vi "STD获取温度校准参数.vi"(7 "探头":T1(ring), 8 "error in (no error)":errorcluster caption="错误输入（无错误）", 11 "MB session in":refnum<class "MB_Master.lvclass">) -> (0 "error out":errorcluster caption="错误输出", 2 "输出值":cluster{"K":sgl, "B":sgl}, 3 "MB session out":refnum<class "MB_Master.lvclass">)   [LabVIEW 2016, in "斯坦道多参数.lvlib"]
uses:
  <vilib>/Plasmionique/MB Master/MB_Master/MB_Master.lvclass
  <vilib>/Plasmionique/MB Master/MB Master.lvlib
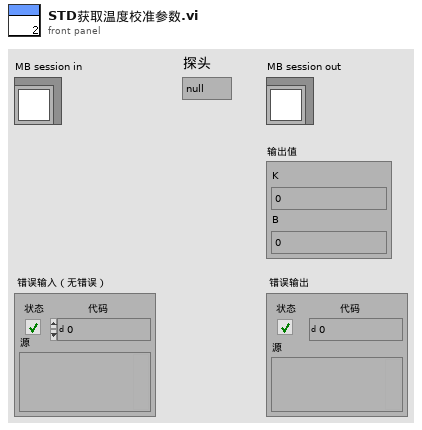
[diagram p1: front panel]
types:
  T1 = enum16{"null", "pH", "DO", "浊度", "电导率", "叶绿素a", "DO2", "藻密度", "悬浮物"}
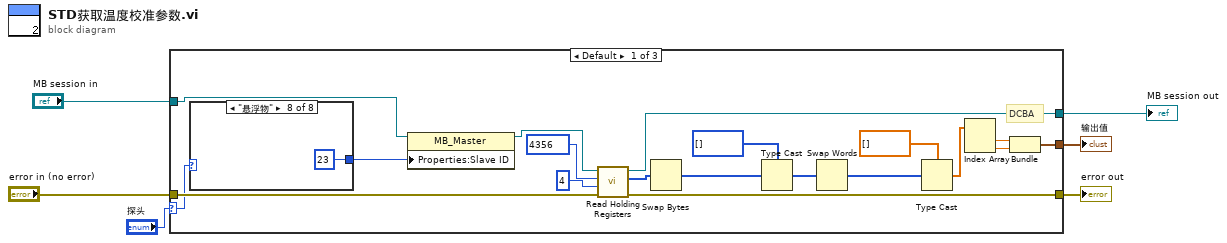
[diagram p0: block diagram]
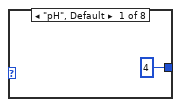
[diagram p2: hidden frame]
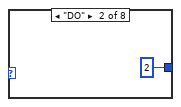
[diagram p3: hidden frame]
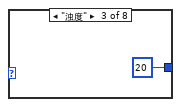
[diagram p4: hidden frame]
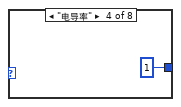
[diagram p5: hidden frame]
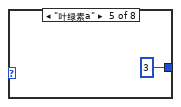
[diagram p6: hidden frame]
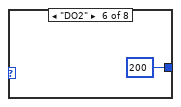
[diagram p7: hidden frame]
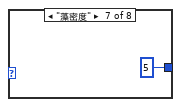
[diagram p8: hidden frame]
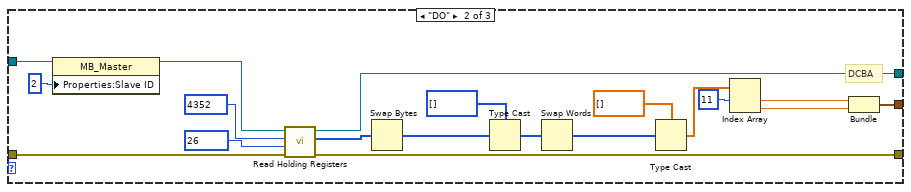
[diagram p9: hidden frame]
diagram:
  n1 = case shown="Default" "探头" {
    selector: "探头" -> [w9 _ _]
    tunnel: "error in (no error)" -> [w16 w43 w53]
    tunnel: [w14 w41 w53] -> w5
    tunnel: "MB session in" -> [w12 w39 w54]
    tunnel: [w11 w38 w54] -> w3
    tunnel: [w8 w36 _] -> w1
    frame Default {
      # "DCBA"
      n2 = case shown="\"悬浮物\"" w9 {
        tunnel: [u16 4 ("y") u16 2 ("y") u16 20 ("y") u16 1 ("y") u16 3 ("y") u16 200 ("y") u16 5 ("y") u16 23 ("y")] -> w10
        frame "pH", Default {
        }
        frame "DO" {
        }
        frame "浊度" {
        }
        frame "电导率" {
        }
        frame "叶绿素a" {
        }
        frame "DO2" {
        }
        frame "藻密度" {
        }
        frame "悬浮物" {
        }
      }
      n3 = property class="MB_Master"(reference=w12, "Properties:Slave ID"=w10) -> (reference out=w15:refnum<class "MB_Master.lvclass">)  [unwired: 1 in, 1 out]
      n4 = call <vilib>:"Read Holding Registers.vi"("error in (no error)"=w16, "quantity"=u16 4, "starting address"=u16 4356, "MB session in"=w15) -> ("error out"=w14:errorcluster, "Registers"=w13:u16[], "MB session out"=w11:refnum<class "MB_Master.lvclass">)  [unwired: 5 in]
      n5 = Swap Bytes(anything=w13) -> (byte swapped=w7:u16[])
      n6 = Type Cast(type=u32[] [] ("数组 2"), x=w7) -> (*(type *) &x=w21:u32[])
      n7 = Swap Words(1:w21) -> (0:w23:u32[])
      n8 = Type Cast(type=sgl[] [] ("数组 2"), x=w23) -> (*(type *) &x=w19:sgl[])
      n9 = Index Array(array=w19) -> (element #1=w18:sgl, element #2=w17:sgl)  [unwired: 2 in]
      n10 = Bundle("数值"=w18, "数值"=w17) -> (w8:cluster{"数值":sgl, "数值":sgl})  [unwired: 1 in]
    }
    frame "DO" {
      # "DCBA"
      n11 = property class="MB_Master"(reference=w39, "Properties:Slave ID"=u16 2 ("y")) -> (reference out=w42:refnum<class "MB_Master.lvclass">)  [unwired: 1 in, 1 out]
      n12 = call <vilib>:"Read Holding Registers.vi"("error in (no error)"=w43, "quantity"=u16 26, "starting address"=u16 4352, "MB session in"=w42) -> ("error out"=w41:errorcluster, "Registers"=w40:u16[], "MB session out"=w38:refnum<class "MB_Master.lvclass">)  [unwired: 5 in]
      n13 = Swap Bytes(anything=w40) -> (byte swapped=w35:u16[])
      n14 = Type Cast(type=u32[] [] ("数组 2"), x=w35) -> (*(type *) &x=w48:u32[])
      n15 = Swap Words(1:w48) -> (0:w50:u32[])
      n16 = Type Cast(type=sgl[] [] ("数组 2"), x=w50) -> (*(type *) &x=w46:sgl[])
      n17 = Index Array(array=w46, index #1=11 ("索引")) -> (element #1=w45:sgl, element #2=w44:sgl)  [unwired: 1 in]
      n18 = Bundle("数值"=w45, "数值"=w44) -> (w36:cluster{"数值":sgl, "数值":sgl})  [unwired: 1 in]
    }
    frame "null" {
    }
  }
  "error out" <- w5
  "MB session out" <- w3
  "输出值" <- w1
